vi "Queue_Driver.vi"(0 "State_In":string, 2 "Queue_Name":string, 5 "State_In_N":string[](array[string]), 7 "Timeout ms (-1)":i32, 11 "Error_In":errorcluster, 13 "Queue_Operation_Select":T1=enum."Dequeue") -> (4 "State_Out":string="Exit", 15 "Error_Out":errorcluster)   [LabVIEW 2021]
doc: "Used to send the imformation of states from one loop to another."
uses:
  Controls/Queue_Operation_Select.ctl
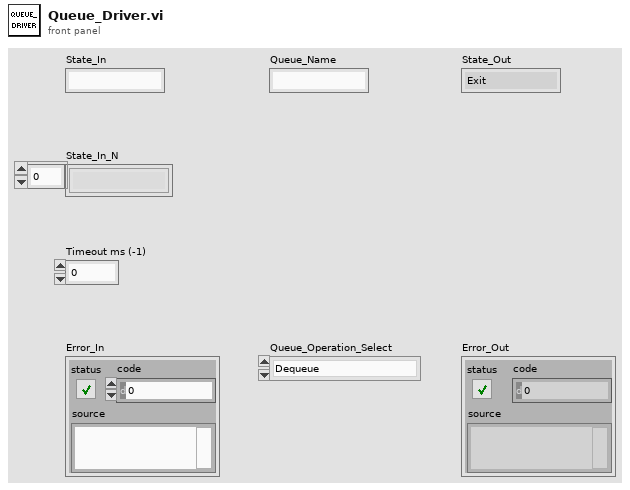
[diagram p1: front panel]
types:
  T1 = typedef "Queue_Operation_Select.ctl" = enum16{"Obtain_Queue", "Enqueue", "Enqueue_at_First", "Enqueue_N", "Dequeue", "Flush_Queue", "Release_Queue"}
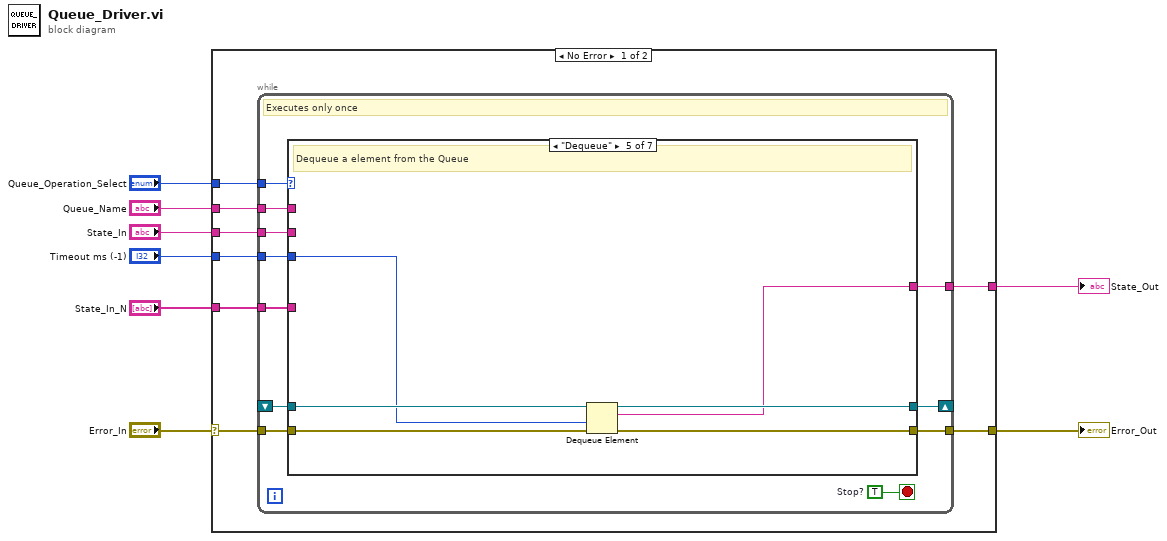
[diagram p0: block diagram]
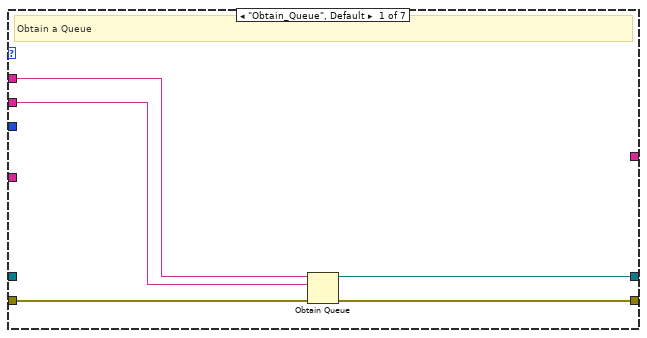
[diagram p2: hidden frame]
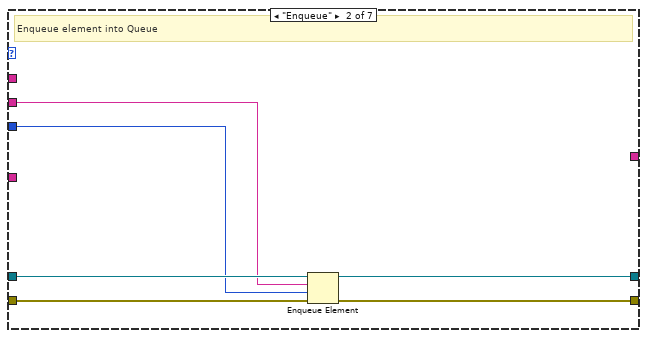
[diagram p3: hidden frame]
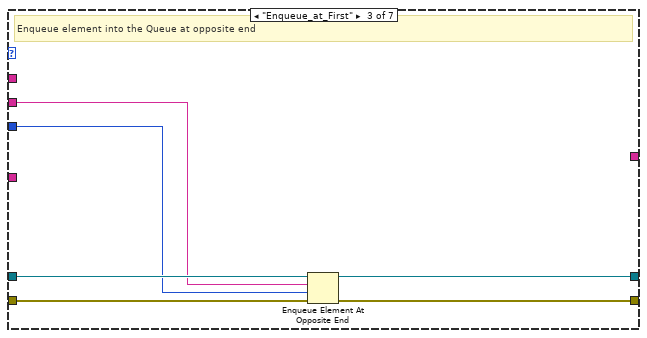
[diagram p4: hidden frame]
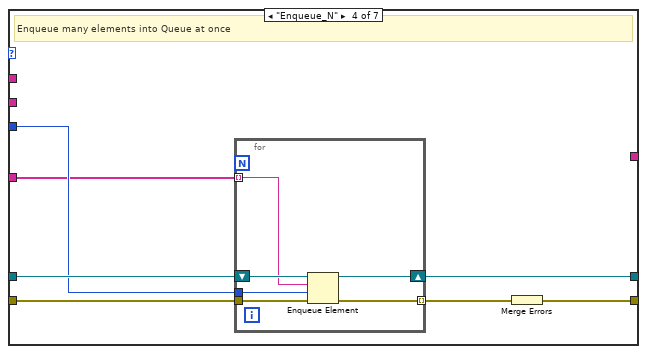
[diagram p5: hidden frame]
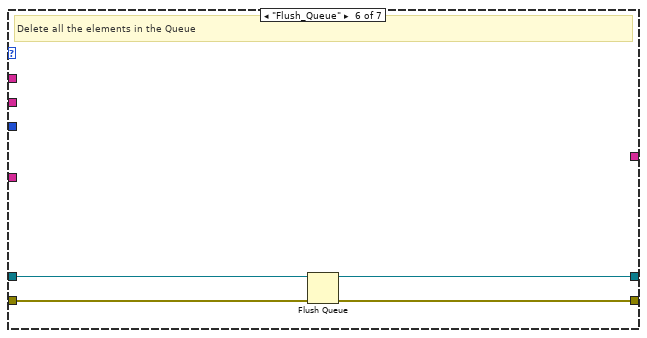
[diagram p6: hidden frame]
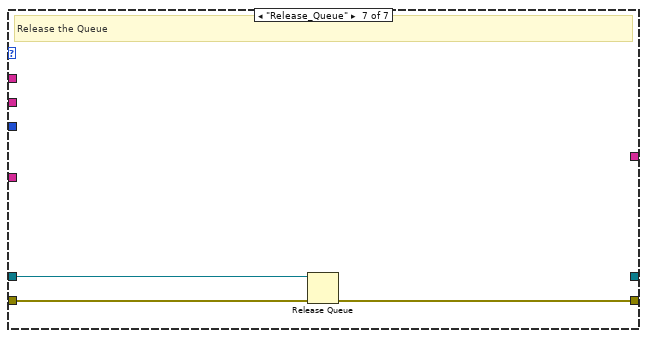
[diagram p7: hidden frame]
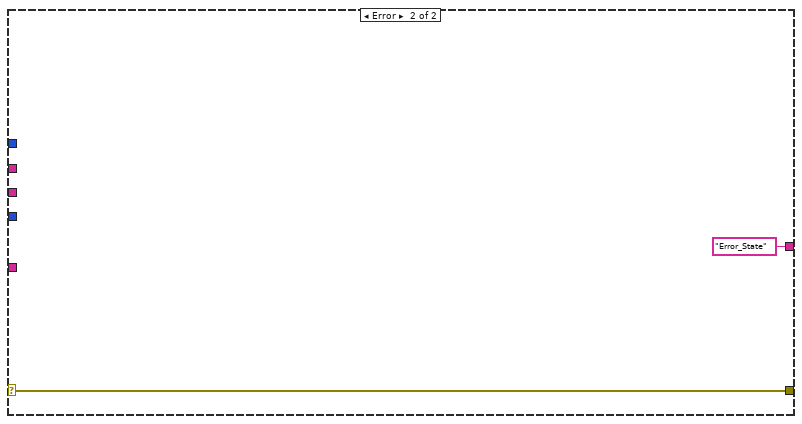
[diagram p8: hidden frame]
diagram:
  n1 = case shown="No Error" "Error_In" {
    selector: "Error_In" -> [w9 w72]
    tunnel: [w16 w72] -> w8
    tunnel: "Queue_Operation_Select" -> [w15 _]
    tunnel: "Queue_Name" -> [w14 _]
    tunnel: "State_In" -> [w13 _]
    tunnel: "Timeout ms (-1)" -> [w12 _]
    tunnel: "State_In_N" -> [w11 _]
    tunnel: [w10 "Error_State" ("State_In")] -> w2
    frame No Error {
      n2 = while {
        tunnel: w9 -> [w27]
        tunnel: [w26] -> w16
        tunnel: w15 -> [w25]
        tunnel: w14 -> [w24]
        tunnel: w13 -> [w23]
        shift-right: [w22] -> _
        shift-left: _ -> [w21]
        tunnel: w12 -> [w20]
        tunnel: w11 -> [w19]
        tunnel: [w18] -> w10
        stop <- w17 stop-if-true
        w17 = TRUE  # Stop?
        # "Executes only once"
        n3 = case shown="\"Dequeue\"" w25 {
          tunnel: [w31 w37 w43 w45 w62 w66 w69] -> w26
          tunnel: w27 -> [w32 w38 w44 w51 w63 w67 w70]
          tunnel: w24 -> [w30 _ _ _ _ _ _]
          tunnel: w23 -> [w29 w35 w41 _ _ _ _]
          tunnel: [w28 w34 w39 w47 w59 w64 _] -> w22
          tunnel: w21 -> [_ w36 w42 w49 w61 w65 w68]
          tunnel: w20 -> [_ w33 w40 w48 w60 _ _]
          tunnel: w19 -> [_ _ _ w46 _ _ _]
          tunnel: [_ _ _ _ w58 _ _] -> w18
          frame "Obtain_Queue", Default {
            # "Obtain a Queue"
            n4 = Obtain Queue(name (unnamed)=w30, element data type=w29, error in (no error)=w32) -> (queue out=w28:refnum<queue>, error out=w31:errorcluster)  [unwired: 2 in, 1 out]
          }
          frame "Enqueue" {
            # "Enqueue element into Queue"
            n5 = Enqueue Element(queue=w36, element=w35, timeout in ms (-1)=w33, error in (no error)=w38) -> (queue out=w34:refnum<queue>, error out=w37:errorcluster)  [unwired: 1 out]
          }
          frame "Enqueue_at_First" {
            # "Enqueue element into the Queue at opposite end"
            n6 = Enqueue Element At Opposite End(queue=w42, element=w41, timeout in ms (-1)=w40, error in (no error)=w44) -> (queue out=w39:refnum<queue>, error out=w43:errorcluster)  [unwired: 1 out]
          }
          frame "Enqueue_N" {
            # "Enqueue many elements into Queue at once"
            n7 = for {
              tunnel: w48 -> [w54]
              shift-right: [w53] -> w47
              shift-left: w49 -> [w55]
              tunnel: w46 -> [w52] mode=indexing
              tunnel: w51 -> [w57]
              tunnel: [w56] -> w50 mode=indexing
              n8 = Enqueue Element(queue=w55, element=w52, timeout in ms (-1)=w54, error in (no error)=w57) -> (queue out=w53:refnum<queue>, error out=w56:errorcluster)  [unwired: 1 out]
            }
            n9 = Merge Errors(w50) -> (w45:errorcluster)
          }
          frame "Dequeue" {
            # "Dequeue a element from the Queue"
            n10 = Dequeue Element(queue=w61, timeout in ms (-1)=w60, error in (no error)=w63) -> (queue out=w59:refnum<queue>, element=w58:string, error out=w62:errorcluster)  [unwired: 1 out]
          }
          frame "Flush_Queue" {
            # "Delete all the elements in the Queue"
            n11 = Flush Queue(queue=w65, error in (no error)=w67) -> (queue out=w64:refnum<queue>, error out=w66:errorcluster)  [unwired: 1 out]
          }
          frame "Release_Queue" {
            # "Release the Queue"
            n12 = Release Queue(queue=w68, error in (no error)=w70) -> (error out=w69:errorcluster)  [unwired: 1 in, 2 out]
          }
        }
      }
    }
    frame Error {
    }
  }
  "Error_Out" <- w8
  "State_Out" <- w2
